vi "11_NOV_VARY_V_GET_I_FOR_LOOP.vi"() -> ()   [LabVIEW 2020]
uses:
  <instrlib>/Agilent B2900 Series/Agilent B2900 Series.lvlib
panel:
  out "SCPI COMMAND":string
  out "XY Graph":cluster{"X":dbl[], "Y":dbl[]}[](graph)
  out "Waveform Chart":dbl(graph)
  out "Measured Current (A)":dbl
  in  "SELECT DEVICE":refnum<visa-resource-name>="USB0::0x0957::0x8E18::MY51140695::INSTR"
  in  "Channel":enum16{"Not Selected", "1", "2"}(ring)
  out "Source Voltage (V)":dbl
  out "Resolution (V)":dbl format="%#_6f"
  in  "Specify number of steps":dbl
  in  "Set final voltage(V)":dbl
  in  "Set initial voltage(V)":dbl
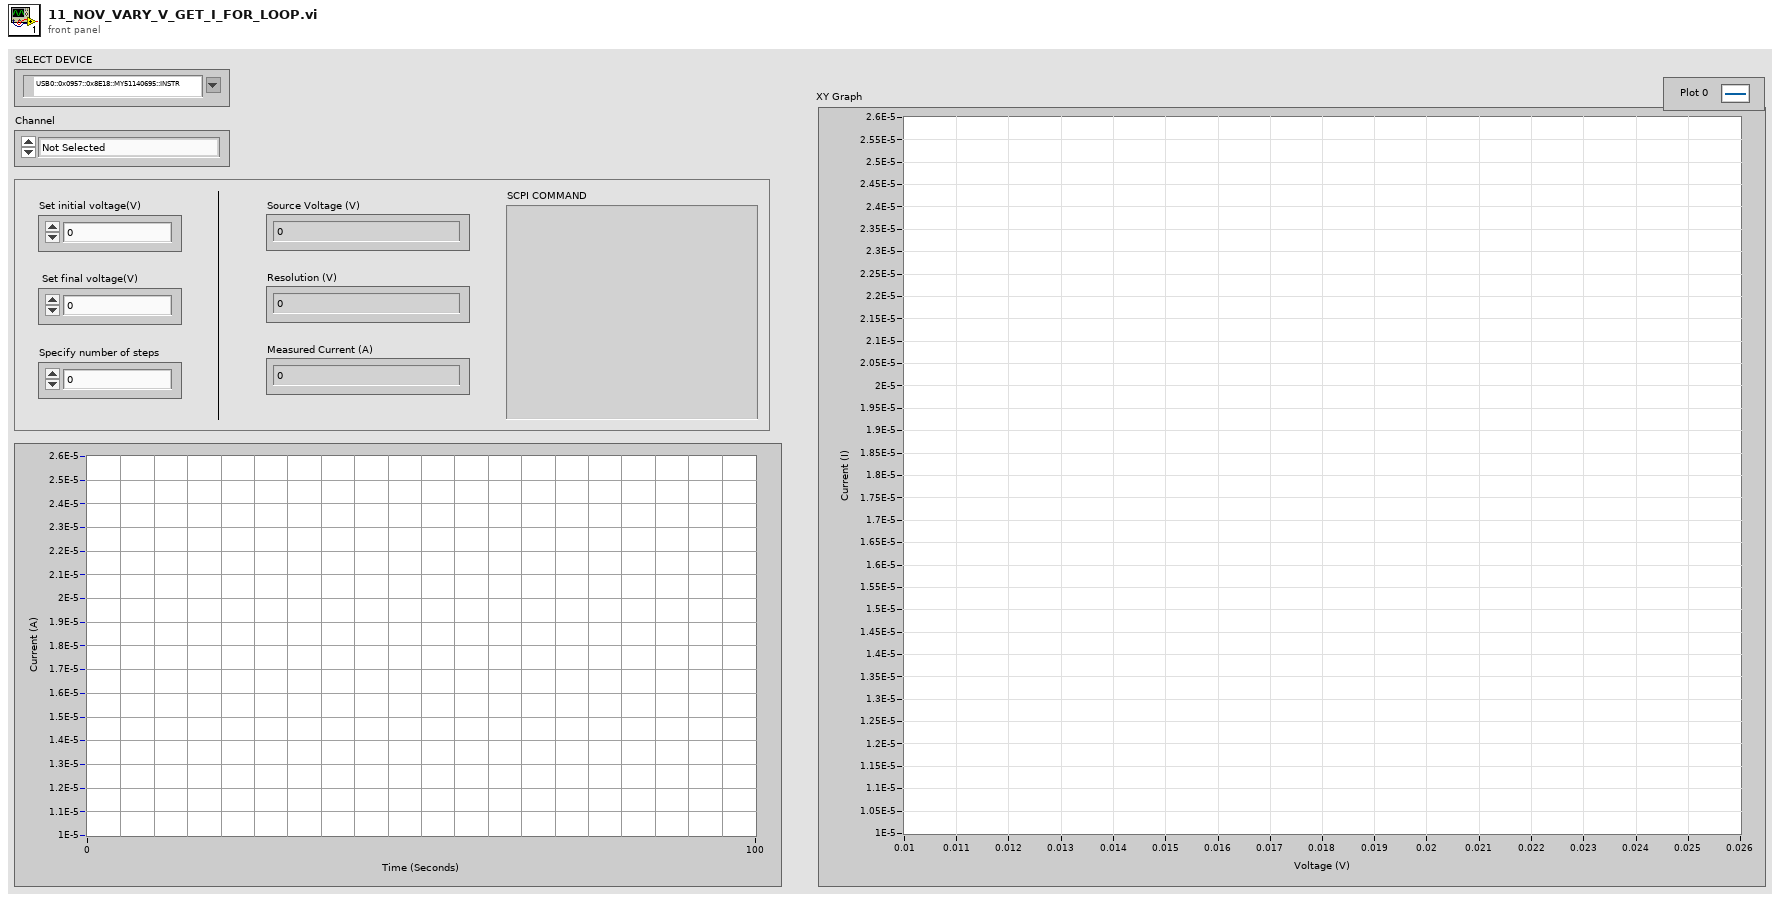
[diagram p1: front panel]
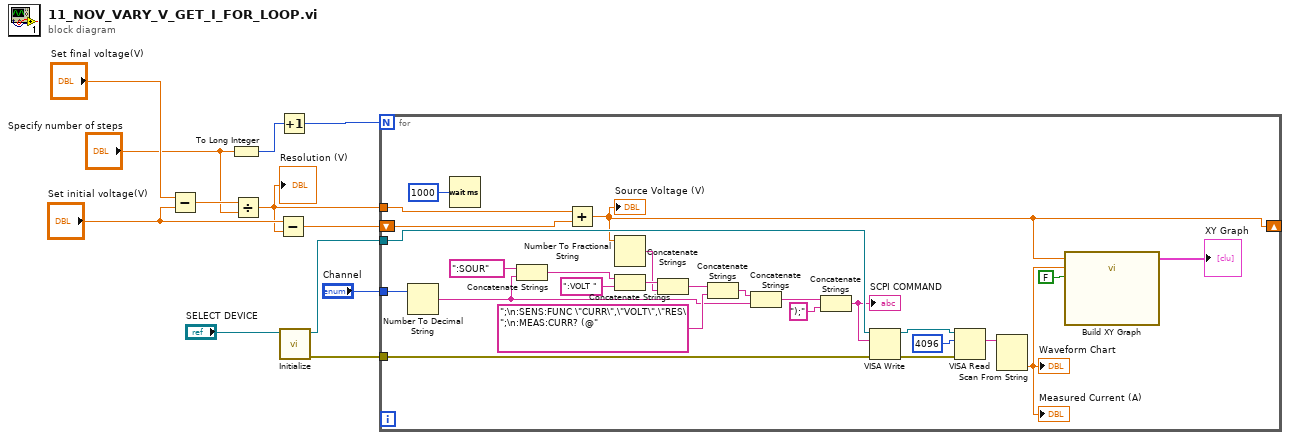
[diagram p0: block diagram]
diagram:
  n1 = Subtract(x="Set final voltage(V)", y="Set initial voltage(V)") -> (x-y=w11:dbl)
  n2 = To Long Integer(number="Specify number of steps") -> (32bit integer=w6:i32)
  n3 = Divide(x=w11, y="Specify number of steps") -> (x/y=w8:dbl)
  "Resolution (V)" <- w8
  n4 = Subtract(x="Set initial voltage(V)", y=w8) -> (x-y=w7:dbl)
  n5 = Increment(x=w6) -> (x+1=w5:i32)
  n6 = call <instrlib>:"Initialize.vi"("VISA resource name"="SELECT DEVICE") -> ("error out"=w1:errorcluster, "VISA resource name out"=w2:refnum<visa-resource-name>)  [unwired: 9 in]
  n7 = for {
    N: w5 -> [_]
    shift-right: [w17] -> _
    shift-left: w7 -> [w38]
    tunnel: w8 -> [w37]
    tunnel: "Channel" -> [w34]
    tunnel: w2 -> [w19]
    tunnel: w1 -> [w18]
    n8 = Number To Decimal String(number=w34) -> (decimal integer string=w24:string)  [unwired: 1 in]
    n9 = Wait (ms)(milliseconds to wait=u32 1000) -> ()  [unwired: 1 out]
    n10 = Concatenate Strings(":SOUR", w24) -> (w33:string)
    n11 = Add(x=w37, y=w38) -> (x+y=w17:dbl)
    "Source Voltage (V)" <- w17
    n12 = Number To Fractional String(number=w17) -> (F-format string=w30:string)  [unwired: 3 in]
    n13 = Concatenate Strings(w33, ":VOLT ") -> (w31:string)
    n14 = Concatenate Strings(w31, w30) -> (w26:string)
    n15 = Concatenate Strings(w26, ";\n:SENS:FUNC \"CURR\",\"VOLT\",\"RES\";\n:MEAS:CURR? (@") -> (w27:string)
    n16 = Concatenate Strings(w27, w24) -> (w28:string)
    n17 = Concatenate Strings(w28, ");" ("string")) -> (w13:string)
    "SCPI COMMAND" <- w13
    n18 = VISA Write(VISA resource name=w19, write buffer=w13, error in (no error)=w18) -> (VISA resource name out=w23:refnum<visa-resource-name>, error out=w22:errorcluster)  [unwired: 1 out]
    n19 = VISA Read(VISA resource name=w23, byte count=u32 4096, error in (no error)=w22) -> (read buffer=w20:string)  [unwired: 3 out]
    n20 = Scan From String(input string=w20) -> (output 1=w16:dbl)  [unwired: 4 in, 3 out]
    "Measured Current (A)" <- w16
    "Waveform Chart" <- w16
    n21 = call "Build XY Graph"("Reset"=FALSE, "Y Input"=w16, "X Input"=w17) -> ("XY Graph"=→"XY Graph":cluster{"X":dbl[], "Y":dbl[]}[])  [unwired: 7 in, 1 out]
  }
